vi "TEST optimize swerve.vi"() -> ()   [LabVIEW 2023]
uses:
  <vilib>/Analysis/coordinate.llb/Angle Units.ctl
  <vilib>/Analysis/coordinate.llb/Angle Range (Degree).ctl
  <vilib>/Analysis/coordinate.llb/Wrap Angle (scalar).vi
  <vilib>/Analysis/NI_AAL_Angle.lvlib
panel:
  out "delta = target - POS":dbl[](array[numeric])
  out "POS":dbl[](array[numeric])
  out "output":T1(array[cluster]) {"+CCW/-CW" format="%_4f"; "ABS out" format="%_4f"; "velocity out" format="%_3f"; "POS out" format="%_4f"}
  in  "input":T2(array[cluster])=[{"POS"=91.0, "target angle"=-1.0, "velocity"=1.0}, {"POS"=0.0, "target angle"=180.0, "velocity"=1.0}, {"POS"=0.0, "target angle"=0.0, "velocity"=0.015}, {"POS"=350.0, "target angle"=0.0, "velocity"=0.015}] {"velocity" format="%_4f"; "target angle" format="%_4f"; "POS" format="%_4f"}
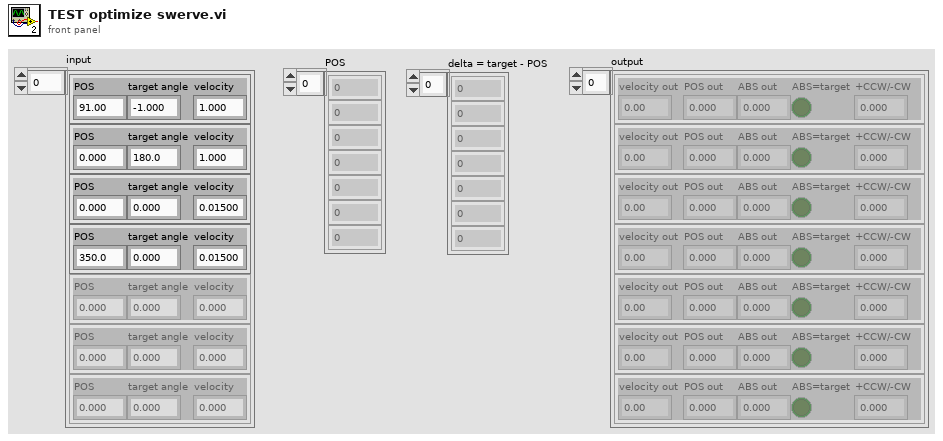
[diagram p1: front panel]
types:
  T1 = cluster{"velocity out":dbl, "POS out":dbl, "ABS out":dbl, "ABS=target":bool, "+CCW/-CW":dbl}[]
  T2 = cluster{"POS":dbl, "target angle":dbl, "velocity":dbl}[]
  T3 = typedef "NI_AAL_Angle.lvlib/Angle Range (Degree).ctl" = u16
  T4 = typedef "NI_AAL_Angle.lvlib/Angle Units.ctl" = i32
  T5 = cluster{"velocity out":dbl, "POS out":dbl, "ABS out":dbl, "ABS=target?":bool, "deg CCW":dbl}
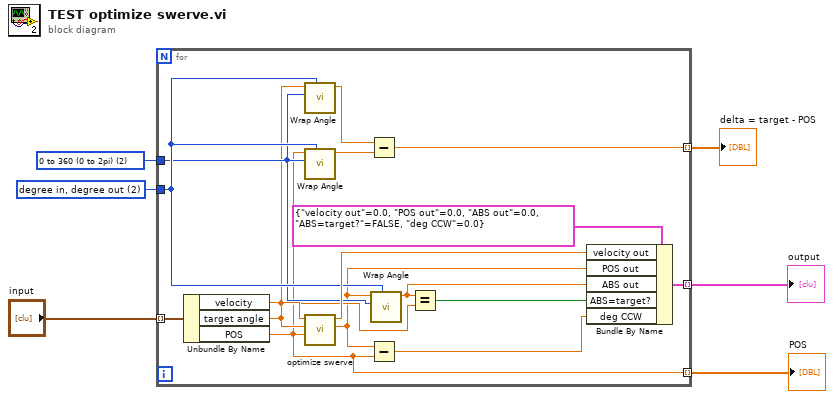
[diagram p0: block diagram]
diagram:
  w4 = T3 2 items=["none", "-180 to 180 (-pi to pi)", "0 to 360 (0 to 2pi)"] ("angle range")
  w3 = T4 2 items=["radian in, radian out", "radian in, degree out", "degree in, degree out", "degree in, radian out"] ("angle units")
  n1 = for {
    tunnel: "input" -> [w22] mode=indexing
    tunnel: [w18] -> w5 mode=indexing
    tunnel: w4 -> [w16]
    tunnel: w3 -> [w17]
    tunnel: [w8] -> w2 mode=indexing
    tunnel: [w15] -> w1 mode=indexing
    n2 = Unbundle By Name(w22) -> ("velocity"=w21:dbl, "target angle"=w11:dbl, "POS"=w8:dbl)
    n3 = call-poly <vilib>:"Wrap Angle.vi"("angle units"=w17, "angle range"=w16, "angle in"=w11) -> ("angle out"=w14:dbl)  [unwired: 7 in, 1 out]
    n4 = call-poly <vilib>:"Wrap Angle.vi"("angle units"=w17, "angle range"=w16, "angle in"=w8) -> ("angle out"=w13:dbl)  [unwired: 7 in, 1 out]
    n5 = call "optimize swerve.vi"("current angle (deg)"=w8, "target angle (deg)"=w11, "velocity"=w21) -> ("steer angle (deg)"=w7:dbl, "velocity"=w19:dbl)  [unwired: 5 in, 2 out]
    n6 = Subtract(x=w14, y=w13) -> (x-y=w15:dbl)
    n7 = Subtract(x=w7, y=w8) -> (x-y=w10:dbl)
    n8 = call-poly <vilib>:"Wrap Angle.vi"("angle units"=w17, "angle range"=w16, "angle in"=w7) -> ("angle out"=w9:dbl)  [unwired: 7 in, 1 out]
    n9 = Equal?(x=w9, y=w11) -> (x = y?=w12:bool)
    n10 = Bundle By Name(cluster=T5 {"velocity out"=0.0, "POS out"=0.0, "ABS out"=0.0, "ABS=target?"=FALSE, "deg CCW"=0.0}, "velocity out"=w19, "POS out"=w7, "ABS out"=w9, "ABS=target?"=w12, "deg CCW"=w10) -> (w18:T5)
  }
  "output" <- w5
  "POS" <- w2
  "delta = target - POS" <- w1
